vi "Get Folder Items.vi"(7 "Calling VI Ref":refnum<vi>, 8 "error in (no error)":errorcluster, 11 "Folder Path":path) -> (0 "error out":errorcluster, 2 "Cancelled?":bool, 3 "Item Data":refnum<class "Item.lvclass">[](array[class]))   [LabVIEW 2020, in "VI Properties Editor.lvlib"]
doc: "Gets all VI data from a folder located at <B>Path</B>."
uses:
  VI Properties Editor.lvlib
  Classes/Item/Item.lvclass
  Classes/Support/Item Type.ctl
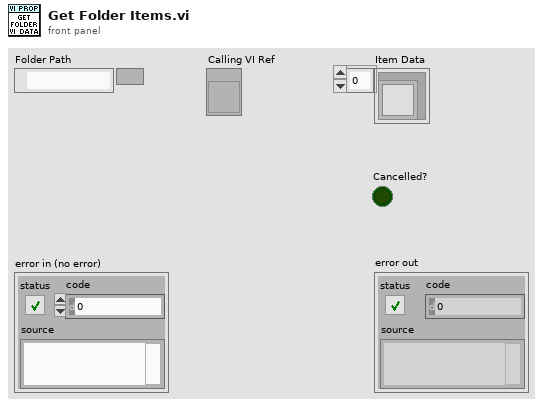
[diagram p1: front panel]
types:
  T1 = typedef "VI Properties Editor.lvlib/Item Type.ctl" = enum16{"Generic", "VI"}
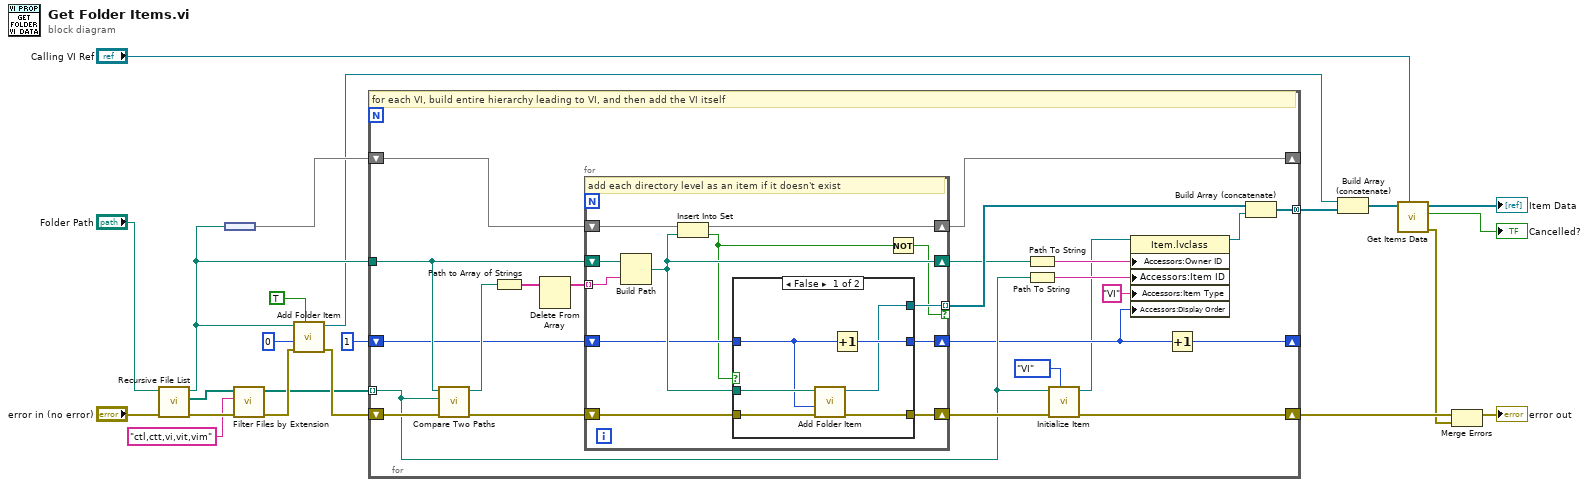
[diagram p0: block diagram]
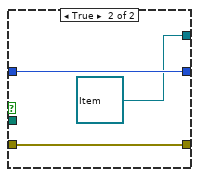
[diagram p2: hidden frame]
diagram:
  n1 = call <vilib>:"Recursive File List.vi"("error in (no error)"="error in (no error)", "Folder Path"="Folder Path") -> ("error out"=w19:errorcluster, "All Files in Dir"=w13:path[], "dup Folder Path"=w9:path)  [unwired: 5 in, 2 out]
  n2 = node(w9) -> (w8:set{path})
  n3 = call "Filter Files by Extension.vi"("error in (no error)"=w19, "Extensions"="ctl,ctt,vi,vit,vim", "Files"=w13) -> ("error out"=w18:errorcluster, "Files out"=w10:path[])  [unwired: 7 in]
  n4 = call "Add Folder Item.vi"("Top-Level? (F)"=TRUE, "error in (no error)"=w18, "Order"=0, "Folder"=w9) -> ("error out"=w17:errorcluster, "Item"=w5:refnum<class "Item.lvclass">)  [unwired: 6 in]
  n5 = for {
    shift-right: [w42] -> w21
    shift-left: w17 -> [w45]
    tunnel: w10 -> [w29] mode=indexing
    tunnel: [w30] -> w6 mode=concatenating
    tunnel: w9 -> [w37]
    shift-right: [w34] -> _
    shift-left: w8 -> [w36]
    shift-right: [w33] -> _
    shift-left: 1 ("Order") -> [w35]
    # "for each VI, build entire hierarchy leading to VI, and then add the VI itself"
    n6 = call <vilib>:"Compare Two Paths.vi"("error in (no error)"=w45, "Path 2"=w29, "Path 1"=w37) -> ("error out"=w44:errorcluster, "Relative Path from 1 to 2"=w41:path)  [unwired: 5 in, 2 out]
    n7 = Path to Array of Strings(0:w41) -> (2:w40:string[])  [unwired: 1 out]
    n8 = Delete From Array(array=w40) -> (array with subset deleted=w39:string[])  [unwired: 2 in, 1 out]
    n9 = for {
      tunnel: w39 -> [w54] mode=indexing
      shift-right: [w53] -> w28
      shift-left: w37 -> [w55]
      shift-right: [w51] -> w34
      shift-left: w36 -> [w52]
      shift-right: [w49] -> w24
      shift-left: w35 -> [w50]
      shift-right: [w56] -> w43
      shift-left: w44 -> [w57]
      tunnel: [w48] -> w32 mode=indexing if=w47
      # "add each directory level as an item if it doesn't exist"
      n10 = Build Path(base path=w55, name or relative path=w54) -> (appended path=w53:path)
      n11 = Insert Into Set(10:w53, 11:w52) -> (2:w46:bool, 3:w51:set{path})
      n12 = case shown="False" w46 {
        tunnel: w57 -> [w63 w66]
        tunnel: w53 -> [w61 _]
        tunnel: w50 -> [w60 w65]
        tunnel: [w59 w65] -> w49
        tunnel: [w62 w66] -> w56
        tunnel: [w58 refnum<class "Item.lvclass"> refnum ("Item")] -> w48
        frame False {
          n13 = call "Add Folder Item.vi"("error in (no error)"=w63, "Order"=w60, "Folder"=w61) -> ("error out"=w62:errorcluster, "Item"=w58:refnum<class "Item.lvclass">)  [unwired: 7 in]
          n14 = Increment(x=w60) -> (x+1=w59:i32)
        }
        frame True {
        }
      }
      n15 = Not(x=w46) -> (.not. x?=w47:bool)
    }
    n16 = Path To String(path=w28) -> (string=w27:string)
    n17 = Path To String(path=w29) -> (string=w26:string)
    n18 = call "Initialize Item.vi"("Item Type"=Item_Type."VI", "error in (no error)"=w43, "Path"=w29) -> ("error out"=w42:errorcluster, "Item"=w23:refnum<class "Item.lvclass">)  [unwired: 7 in]
    n19 = property class="Item.lvclass"(reference=w23, "Accessors:Owner ID"=w27, "Accessors:Item ID"=w26, "Accessors:Item Type"="VI" ("Item Type"), "Accessors:Display Order"=w24) -> (reference out=w31:refnum<class "Item.lvclass">)  [unwired: 1 in, 1 out]
    n20 = Increment(x=w24) -> (x+1=w33:i32)
    n21 = Build Array (concatenate)(w32, w31) -> (w30:refnum<class "Item.lvclass">[])
  }
  n22 = Build Array (concatenate)(w5, w6) -> (w4:refnum<class "Item.lvclass">[])
  n23 = call "Get Items Data.vi"("Calling VI Ref"="Calling VI Ref", "Items"=w4) -> ("error out"=w16:errorcluster, "Cancelled?"=→"Cancelled?":bool, "Items out"=→"Item Data":refnum<class "Item.lvclass">[])  [unwired: 7 in]
  n24 = Merge Errors(w21, w16) -> (→"error out":errorcluster)
